vi "GetFrameRate.vi"(8 "error in (no error)":errorcluster, 11 "CameraTestingBL in":refnum<class "CameraTesting.lvclass">) -> (0 "error out":errorcluster, 2 "Frame Rate":T1 items=["30", "60", "120"], 3 "CameraTestingBL out":refnum<class "CameraTesting.lvclass">)   [LabVIEW 2020, in "CameraTesting.lvlib" / "CameraTesting.lvclass"]
doc: "Get the frame rate of the camera"
uses:
  CameraTesting.lvclass
  TypeDef/FrameRate.ctl
  CameraTesting.lvclass/CameraTesting.ctl
  ICamera/ICamera/ICamera.lvclass
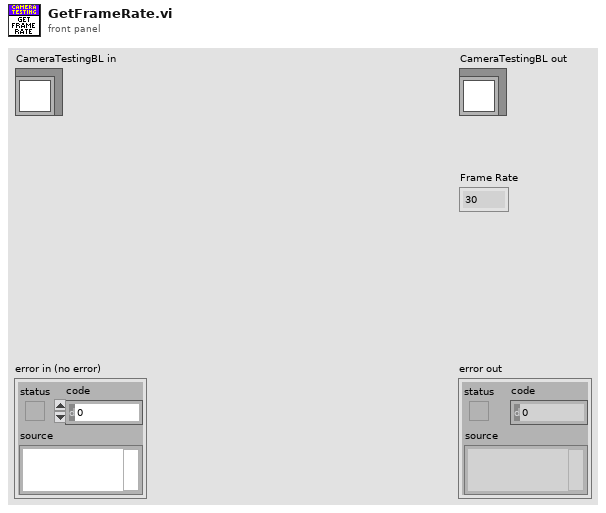
[diagram p1: front panel]
types:
  T1 = typedef "CameraTesting.lvlib/CameraTesting.lvclass/FrameRate.ctl" = u8
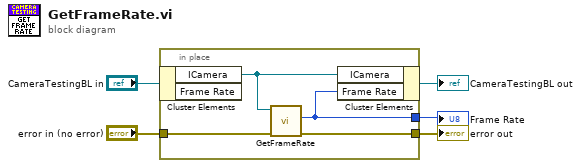
[diagram p0: block diagram]
diagram:
  n1 = in-place {
    in-place-border: "error in (no error)" -> [w9]
    in-place-border: [w6] -> w4
    in-place-border: [w8] -> w3
    n2 = in-place-cluster #1("CameraTestingBL in") -> ("ICamera"=w7:refnum<class "ICamera.lvclass">)  [unwired: 1 out]
    n3 = call-dynamic "GetFrameRate.vi"("error in (no error)"=w9, "ICamera in"=w7) -> ("error out"=w8:errorcluster, "Frame Rate"=w6:u8)  [unwired: 7 in, 1 out]
    n4 = in-place-cluster #1("ICamera"=w7, "Frame Rate"=w6) -> (→"CameraTestingBL out":refnum<class "CameraTesting.lvclass">)
  }
  "error out" <- w3
  "Frame Rate" <- w4
